vi "Instr_InitObject.vi"(8 "error in (no error)":errorcluster, 9 "Instrument Configuration":variant, 10 "Instrument address":refnum<visa-resource-name>, 11 "HP4284A in":refnum<class "HP4284A.lvclass">) -> (0 "error out":errorcluster, 3 "HP4284A out":refnum<class "HP4284A.lvclass">)   [LabVIEW 2018, in "HP4284A.lvclass"]
uses:
  HP4284A.lvclass
  InstrumentSetup.vi
  HP4284A_CommandsGlobal.vi
  LCRControl.lvclass
  InstrControl.lvclass
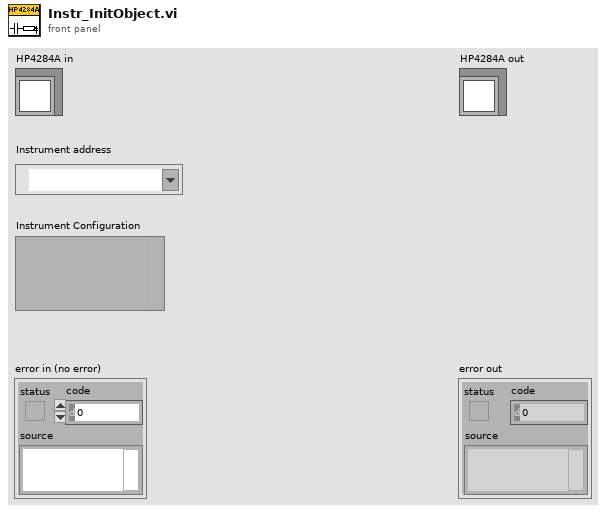
[diagram p1: front panel]
types:
  T1 = cluster{"RC Configuration":u16, "AC amplitude [V]":dbl, "AC frequency [Hz]":i32, "HP 4284A Configurations":cluster{"Consider OC":bool, "Consider SC":bool}}
  T2 = cluster{"Instrument name":string, "Instrument type":u16, "Command \"Initialise LCR\"":string, "Command \"OC Trim\"":string, "Command \"LCR Readout\"":string}
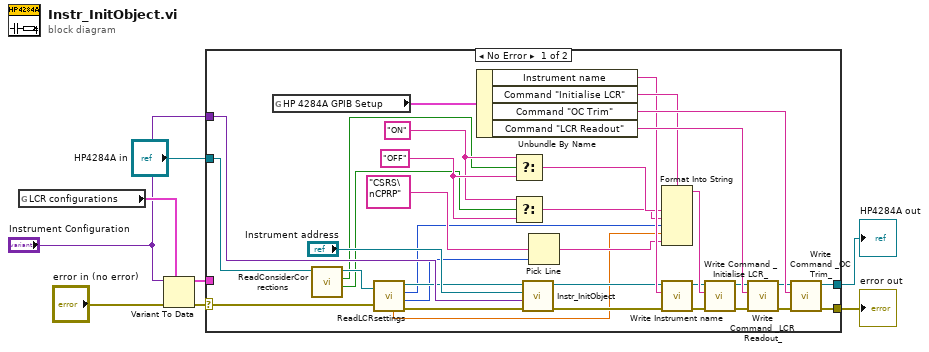
[diagram p0: block diagram]
diagram:
  n1 = global read "InstrumentSetup.vi" "LCR configurations"() -> (w8:T1)
  n2 = Variant To Data(error in="error in (no error)", type=w8, Variant="Instrument Configuration") -> (data=w7:T1, error out=w6:errorcluster)
  n3 = case shown="No Error" w6 {
    selector: w6 -> [w14 w44]
    tunnel: [w37 w44] -> w1
    tunnel: [w38 w43] -> w4
    tunnel: "HP4284A in" -> [w12 w43]
    tunnel: w7 -> [_ _]
    tunnel: "Instrument Configuration" -> [w27 _]
    frame No Error {
      w22 = "OFF"
      w21 = "ON"
      n4 = global read "HP4284A_CommandsGlobal.vi" "HP 4284A GPIB Setup"() -> (w25:T2)
      n5 = call-dynamic "ReadConsiderCorrections.vi"("HP4284A.lvclass in"=w12) -> ("Consider SC"=w10:bool, "Consider OC"=w9:bool, "HP4284A.lvclass  out"=w11:refnum<class "HP4284A.lvclass">)  [unwired: 7 in, 1 out]
      n6 = call-dynamic "ReadLCRsettings.vi"("error in (no error)"=w14, "LCRControl in"=w11) -> ("error out"=w13:errorcluster, "RC Configuration"=w17:u16, "AC frequency [Hz]"=w15:i32, "LCRControl out"=w18:refnum<class "HP4284A.lvclass">, "AC amplitude [V]"=w16:sgl)
      n7 = Unbundle By Name(w25) -> ("Instrument name"=w32:string, "Command \"Initialise LCR\""=w34:string, "Command \"OC Trim\""=w41:string, "Command \"LCR Readout\""=w42:string)
      n8 = Select(t=w21, s=w9, f=w22) -> (s? t:f=w23:string)
      n9 = Select(t=w21, s=w10, f=w22) -> (s? t:f=w20:string)
      n10 = call-parent "Instr_InitObject.vi"("error in (no error)"=w13, "Instrument Configuration"=w27, "Instrument address"="Instrument address", "LCRControl in"=w18) -> ("error out"=w31:errorcluster, "LCRControl out"=w29:refnum<class "HP4284A.lvclass">)  [unwired: 6 in]
      n11 = Pick Line(multi-line string="CSRS\nCPRP", line index=w17) -> (output string=w19:string)  [unwired: 1 in]
      n12 = Format Into String(format string=w34, w23, w20, w15, w16, w19) -> (resulting string=w33:string)  [unwired: 2 in, 1 out]
      n13 = call-dynamic "Write Instrument name.vi"("error in (no error)"=w31, "Instrument name"=w32, "InstControl in"=w29) -> ("error out"=w30:errorcluster, "InstControl out"=w28:refnum<class "HP4284A.lvclass">)  [unwired: 7 in]
      n14 = call-dynamic "Write Command _Initialise LCR_.vi"("error in (no error)"=w30, "Command \"Initialise LCR\""=w33, "LCRControl in"=w28) -> ("error out"=w36:errorcluster, "LCRControl out"=w40:refnum<class "HP4284A.lvclass">)  [unwired: 7 in]
      n15 = call-dynamic "Write Command _LCR Readout_.vi"("error in (no error)"=w36, "Command \"LCR Readout\""=w42, "LCRControl in"=w40) -> ("error out"=w35:errorcluster, "LCRControl out"=w39:refnum<class "HP4284A.lvclass">)  [unwired: 7 in]
      n16 = call-dynamic "Write Command _OC Trim_.vi"("error in (no error)"=w35, "Command \"OC Trim\""=w41, "LCRControl in"=w39) -> ("error out"=w37:errorcluster, "LCRControl out"=w38:refnum<class "HP4284A.lvclass">)  [unwired: 7 in]
    }
    frame Error {
    }
  }
  "error out" <- w1
  "HP4284A out" <- w4
